vi "Filter Test Cases.vi"(8 "error in (no error)":errorcluster, 11 "Classes to Filter":path[](array[path])) -> (0 "error out":errorcluster, 3 "Filtered Classes":path[](array[path]))   [LabVIEW 2020, in "Test Finder.lvclass"]
uses:
  Test Finder.lvclass
  API/LUnit Test Case/LUnit Test Case.lvclass
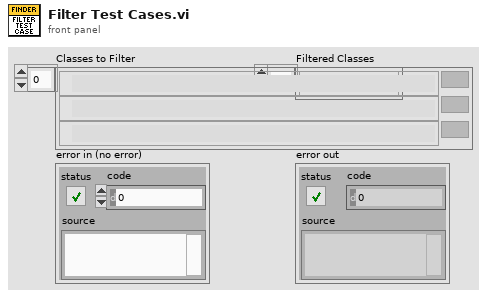
[diagram p1: front panel]
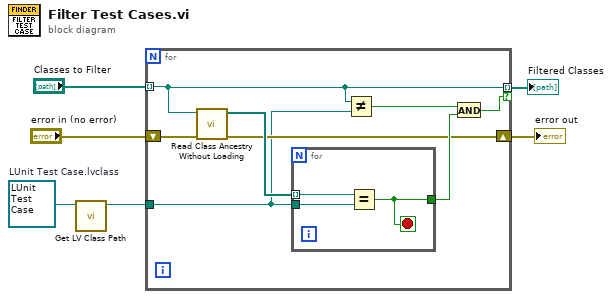
[diagram p0: block diagram]
diagram:
  w3 = refnum<class "LUnit Test Case.lvclass"> refnum  # LUnit Test Case.lvclass
  n1 = call <vilib>:"Get LV Class Path.vi"("object"=w3) -> ("class path"=w2:path)  [unwired: 9 in, 1 out]
  n2 = for {
    tunnel: "Classes to Filter" -> [w10] mode=indexing
    shift-right: [w11] -> w4
    shift-left: "error in (no error)" -> [w14]
    tunnel: w2 -> [w9]
    tunnel: [w10] -> w1 mode=indexing if=w8
    n3 = call <vilib>:"Read Class Ancestry Without Loading.vi"("error in (no error)"=w14, "LabVIEW Class Path"=w10) -> ("error out"=w11:errorcluster, "Class Ancestry"=w13:path[])  [unwired: 8 in]
    n4 = for {
      tunnel: w13 -> [w17] mode=indexing
      tunnel: w9 -> [w16]
      tunnel: [w15] -> w12
      stop <- w15 stop-if-true
      n5 = Equal?(x=w17, y=w16) -> (x = y?=w15:bool)
    }
    n6 = Not Equal?(x=w10, y=w9) -> (x != y?=w7:bool)
    n7 = And(x=w7, y=w12) -> (x .and. y?=w8:bool)
  }
  "Filtered Classes" <- w1
  "error out" <- w4
